vi "SGLtoBase64.vi"(10 "SGL Array":sgl[](array[numeric])) -> (2 "Base64 String":string, 3 "length":i32)   [LabVIEW 2012]
doc: "This VI converts a string to its Base64 equivalent. Base64 strings are commonly used in Internet protocols such as HTTP, SMTP, etc."
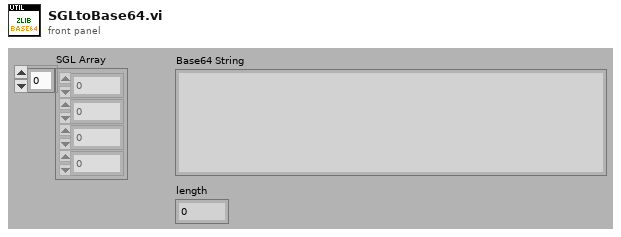
[diagram p1: front panel]
types:
  T1 = enum16{"big-endian, network order", "native, host order", "little-endian"}
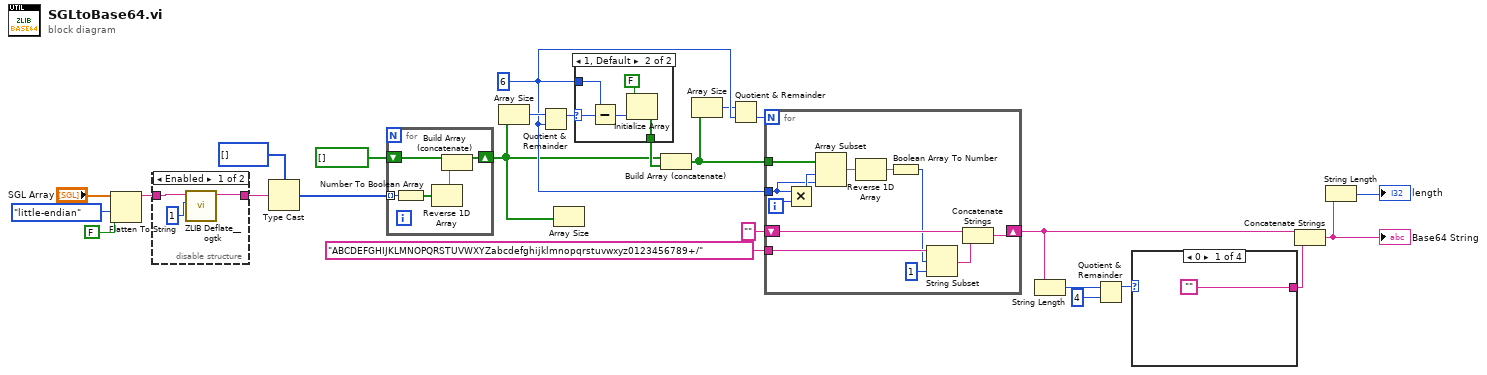
[diagram p0: block diagram]
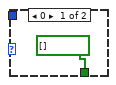
[diagram p3: hidden frame]
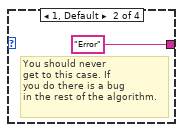
[diagram p4: hidden frame]
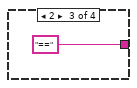
[diagram p5: hidden frame]
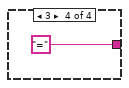
[diagram p6: hidden frame]
diagram:
  w14 = 6 ("y")
  n1 = Flatten To String(anything="SGL Array", prepend array or string size? (T)=FALSE, byte order (0:big-endian, network order)=T1."little-endian") -> (data string=w2:string)  [unwired: 1 in, 2 out]
  n2 = disable-structure shown="Enabled" {
    disable-tunnel: w2 -> [w28 w29]
    disable-tunnel: [w27 w29] -> w1
    frame Enabled {
      n3 = call <userlib>:"ZLIB Deflate__ogtk.vi"("compression level (default)"=1, "input"=w28) -> ("deflated output"=w27:string)  [unwired: 3 in, 2 out]
    }
    frame Disabled {
    }
  }
  n4 = Type Cast(type=u8[] [], x=w1) -> (*(type *) &x=w4:u8[])
  n5 = for {
    tunnel: w4 -> [w34] mode=indexing
    shift-right: [w31] -> w11
    shift-left: bool[] [] -> [w33]
    n6 = Number To Boolean Array(number=w34) -> (Boolean array=w32:bool[])
    n7 = Reverse 1D Array(array=w32) -> (reversed array=w30:bool[])
    n8 = Build Array (concatenate)(w33, w30) -> (w31:bool[])
  }
  n9 = Array Size(array=w11) -> (size(s)=w17:i32)
  n10 = Quotient & Remainder(x=w17, y=w14) -> (x-y*floor(x/y)=w16:i32)  [unwired: 1 out]
  n11 = Array Size(array=w11) -> ()  [unwired: 1 out]
  n12 = case shown="1, Default" w16 {
    selector: w16 -> [_ w39]
    tunnel: [bool[] [] w36] -> w15
    tunnel: w14 -> [_ w38]
    frame 0 {
    }
    frame 1, Default {
      n13 = Subtract(x=w38, y=w39) -> (x-y=w40:i32)
      n14 = Initialize Array(FALSE, w40) -> (w36:bool[])
    }
  }
  n15 = Build Array (concatenate)(w11, w15) -> (w13:bool[])
  n16 = Array Size(array=w13) -> (size(s)=w12:i32)
  n17 = Quotient & Remainder(x=w12, y=w14) -> (floor(x/y)=w18:i32)  [unwired: 1 out]
  n18 = for {
    N: w18 -> [_]
    tunnel: w13 -> [w51]
    tunnel: w14 -> [w49]
    tunnel: "ABCDEFGHIJKLMNOPQRSTUVWXYZabcdefghijklmnopqrstuvwxyz0123456789+/" -> [w48]
    shift-right: [w46] -> w9
    shift-left: "" -> [w45]
    i -> [w52]
    n19 = Multiply(x=w49, y=w52) -> (x*y=w50:i32)
    n20 = Array Subset(array=w51, index=w50, length=w49) -> (w41:bool[])
    n21 = Reverse 1D Array(array=w41) -> (reversed array=w42:bool[])
    n22 = Boolean Array To Number(Boolean array=w42) -> (number=w43:u32)
    n23 = String Subset(string=w48, offset (0)=w43, length (rest)=1 ("length (rest)")) -> (substring=w44:string)
    n24 = Concatenate Strings(w45, w44) -> (w46:string)
  }
  n25 = String Length(string=w9) -> (length=w22:i32)
  n26 = Quotient & Remainder(x=w22, y=4) -> (x-y*floor(x/y)=w20:i32)  [unwired: 1 out]
  n27 = case shown="0" w20 {
    tunnel: ["" "Error" "==" "="] -> w19
    frame 0 {
    }
    frame 1, Default {
      # "You should never\nget to this case. If\nyou do there is a bug\nin the rest of the algorithm."
    }
    frame 2 {
    }
    frame 3 {
    }
  }
  n28 = Concatenate Strings(w9, w19) -> (w5:string)
  "Base64 String" <- w5
  n29 = String Length(string=w5) -> (length=→"length":i32)
